vi "Get Panel Logic.vi"(8 "error in (no error)":errorcluster, 11 "Form Model Configuration in":refnum<class "Form Model Configuration.lvclass">) -> (0 "error out":errorcluster, 2 "Panel Logic":refnum<class "Model Panel Logic.lvclass">, 3 "Form Model Configuration out":refnum<class "Form Model Configuration.lvclass">)   [LabVIEW 2020, in "Form Model Configuration.lvlib" / "Form Model Configuration.lvclass"]
uses:
  Form Model Configuration.lvclass
  Model Panel Logic/Model Panel Logic.lvclass
  Form Model Configuration.lvclass/Form Model Configuration.ctl
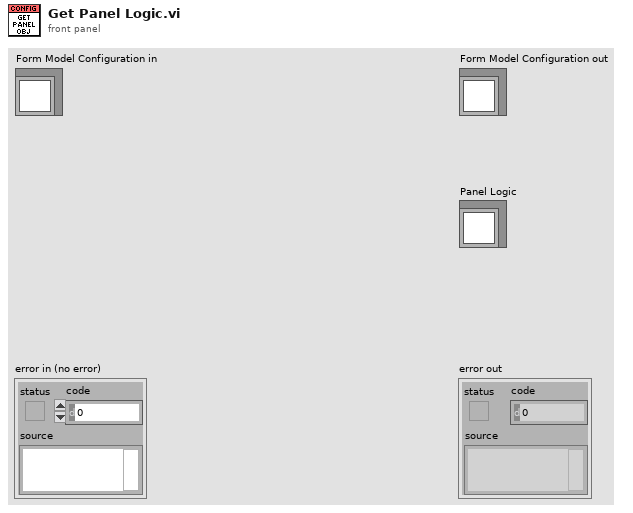
[diagram p1: front panel]
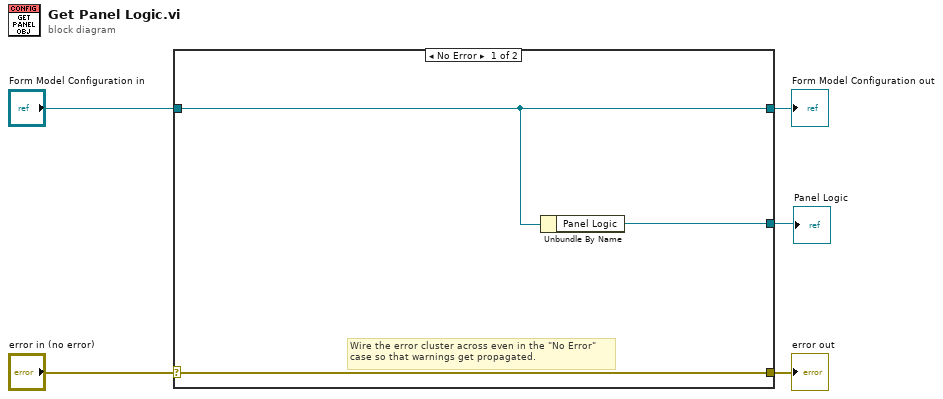
[diagram p0: block diagram]
diagram:
  n1 = case shown="No Error" "error in (no error)" {
    selector: "error in (no error)" -> [w8 w10]
    tunnel: [w8 w10] -> w4
    tunnel: [w7 w9] -> w2
    tunnel: "Form Model Configuration in" -> [w7 w9]
    tunnel: [w6 _] -> w1
    frame No Error {
      # "Wire the error cluster across even in the \"No Error\"\ncase so that warnings get propagated."
      n2 = Unbundle By Name(w7) -> ("Panel Logic"=w6:refnum<class "Model Panel Logic.lvclass">)
    }
    frame Error {
    }
  }
  "error out" <- w4
  "Form Model Configuration out" <- w2
  "Panel Logic" <- w1
